vi "Consume.vi"(8 "error in (no error)":errorcluster, 11 "Alpaca Parser in":refnum<class "Parser.lvclass">) -> (0 "error out":errorcluster, 3 "Alpaca Parser out":refnum<class "Parser.lvclass">)   [LabVIEW 2013, in "JKI JSON Serialization.lvlib" / "Parser.lvclass"]
uses:
  Parser.lvclass
  Parser.lvclass/Parser.ctl
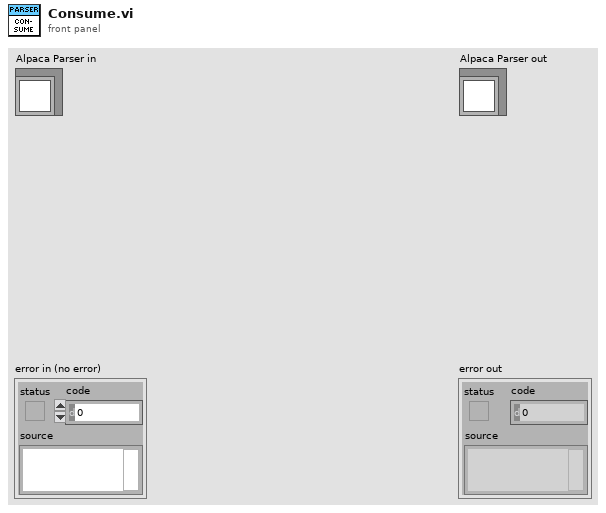
[diagram p1: front panel]
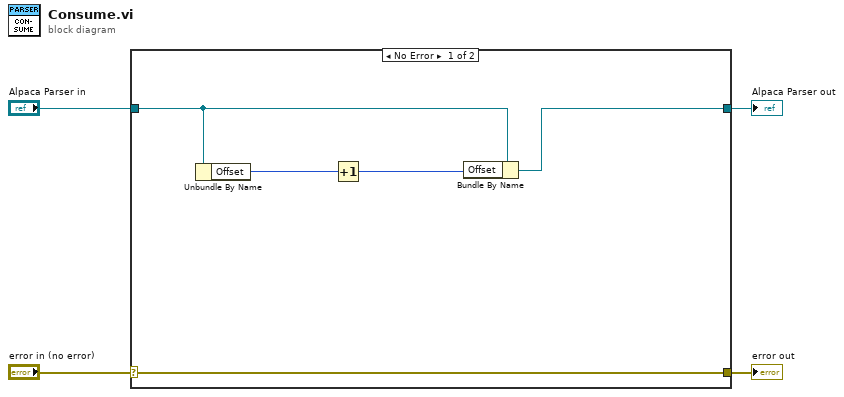
[diagram p0: block diagram]
diagram:
  n1 = case shown="No Error" "error in (no error)" {
    selector: "error in (no error)" -> [w9 w11]
    tunnel: [w9 w11] -> w3
    tunnel: [w5 w10] -> w1
    tunnel: "Alpaca Parser in" -> [w6 w10]
    frame No Error {
      n2 = Unbundle By Name(w6) -> ("Offset"=w8:i32)
      n3 = Increment(x=w8) -> (x+1=w7:i32)
      n4 = Bundle By Name(cluster=w6, "Offset"=w7) -> (w5:refnum<class "Parser.lvclass">)
    }
    frame Error {
    }
  }
  "error out" <- w3
  "Alpaca Parser out" <- w1
